vi "Begin.vi"(8 "error in":errorcluster) -> (0 "error out":errorcluster)   [LabVIEW 2018]
doc: "Called before other user functions, this VI is expected to open initial I/O refnums, load in file data, and do all program initialization. Notice that the <B>error out</B> terminal is simply used for data flow. Wiring it to other structures or subVIs ensures that this VI runs first."
uses:
  <vilib>/Rock Robotics/WPI/SafetyOutput/WPI_SafetyOutputConfigMenu.ctl
  <vilib>/Rock Robotics/WPI/DriverStation/WPI_DriverStationRobotMode2.ctl
  <vilib>/Rock Robotics/WPI/Joystick/WPI_JoystickDeviceEnum.ctl
  <vilib>/Rock Robotics/SystemInterfaces/DIO/FPGA_DIOChannel.ctl
  <vilib>/Rock Robotics/WPI/Solenoid/WPI_SolenoidChannel.ctl
  Robot Global Data.vi
  <vilib>/Rock Robotics/Network Tables/NT Write String Array.vi
  <vilib>/Rock Robotics/WPI/RobotDrive/WPI_RobotDriveOpen4MotorWithExistingMotors.vi
  <vilib>/Rock Robotics/WPI/Counter/WPI_CounterDigitalInputToDigitalSource.vi
  <vilib>/Rock Robotics/WPI/Counter/WPI_CounterOpen UpDown Mode.vi
  <vilib>/Rock Robotics/WPI/Solenoid/WPI_SolenoidOpenDouble.vi
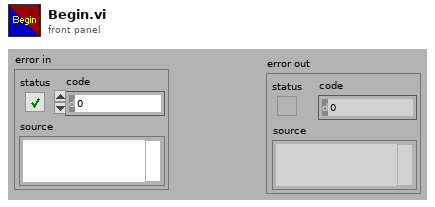
[diagram p1: front panel]
types:
  T1 = typedef "FPGA_DIOChannel.ctl" = enum8{"DIO 0", "DIO 1", "DIO 2", "DIO 3", "DIO 4", "DIO 5", "DIO 6", "DIO 7", "DIO 8", "DIO 9", "DIO MXP 0", "DIO MXP 1", "DIO MXP 2", "DIO MXP 3", "DIO MXP 4", "DIO MXP 5", "DIO MXP 6", "DIO MXP 7", "DIO MXP 8", "DIO MXP 9", "DIO MXP 10", "DIO MXP 11", "DIO MXP 12", "DIO MXP 13", "DIO MXP 14", "DIO MXP 15", "SPI Port CS1", "SPI Port CS2", "SPI Port CS3", "SPI Port MISO", "SPI Port MOSI", "Invalid"}
  T2 = typedef "WPI_SolenoidChannel.ctl" = enum8{"Solenoid 0", "Solenoid 1", "Solenoid 2", "Solenoid 3", "Solenoid 4", "Solenoid 5", "Solenoid 6", "Solenoid 7", "Invalid"}
  T3 = typedef "WPI_JoystickDeviceEnum.ctl" = enum16{"USB 0", "USB 1", "USB 2", "USB 3", "USB 4", "USB 5"}
  T4 = enum16{"Rising Edge", "Falling Edge", "Raising & Falling Edge", "Disabled"}
  T5 = typedef "WPI_DriverStationRobotMode2.ctl" = enum16{"Autonomous Disabled", "Autonomous Enabled", "Teleop Disabled", "Teleop Enabled", "Disconnected", "Finish", "Test Disabled", "Test Enabled", "Emergency Stopped"}
  T6 = typedef "WPI_SafetyOutputConfigMenu.ctl" = enum16{"Enable", "Disable"}
  T7 = typedef "WPI_MotorControlDeviceRef.ctl" = cluster{"DeviceStatus":errorcluster, "Type":T8, "PWM":cluster{"PWM Channel":T9, "DeadBand":T10}, "CAN":cluster{"Device Number":u8, "SetOutput VI Ref":variant, "GetOutput VI Ref":variant, "Enable VI Ref":variant, "Disable VI Ref":variant, "Data":variant}, "Invert":bool, "DIO PWM":cluster{"PWM \"Enable\" Channel":T9, "DIOChannel":T1, "PWM Rate":dbl}}
  T8 = typedef "WPI_MotorControlType.ctl" = enum16{"PWM", "CAN", "DIO PWM"}
  T9 = typedef "FPGA_DIOPWMChannel.ctl" = enum8{"PWM 0", "PWM 1", "PWM 2", "PWM 3", "PWM 4", "PWM 5", "PWM 6", "PWM 7", "PWM 8", "PWM 9", "PWM MXP 0", "PWM MXP 1", "PWM MXP 2", "PWM MXP 3", "PWM MXP 4", "PWM MXP 5", "PWM MXP 6", "PWM MXP 7", "PWM MXP 8", "PWM MXP 9", "Invalid"}
  T10 = typedef "WPI_PWMDeadband.ctl" = cluster{"Name":string, "maxPositivePwm":i32, "minPositivePwm":i32, "centerPwm":i32, "maxNegativePwm":i32, "minNegativePwm":i32, "angularRange":u16}
  T11 = typedef "WPI_DigitalInputDevRef.ctl" = cluster{"DevStatus":errorcluster, "DIO Channel":T1}
  T12 = typedef "WPI_DigitalOutputDevRef.ctl" = cluster{"DIO Channel":T1, "DevStatus":errorcluster}
  T13 = typedef "FPGA_CounterEncoderSourceConvertionLVSourceType.ctl" = cluster{"DevStatus":errorcluster, "AnalogTriggerMode?":bool, "DigitalMode":cluster{"DIO Channel":T14}, "AnalogTriggerMode":cluster{"AnalogTriggerIndex":T15, "OutputType":T16}}
  T14 = typedef "FPGA_DIODigitalSourceChannel.ctl" = enum8{"DIO 0", "DIO 1", "DIO 2", "DIO 3", "DIO 4", "DIO 5", "DIO 6", "DIO 7", "DIO 8", "DIO 9", "DIO MXP 0", "DIO MXP 1", "DIO MXP 2", "DIO MXP 3", "DIO MXP 4", "DIO MXP 5", "DIO MXP 6", "DIO MXP 7", "DIO MXP 8", "DIO MXP 9", "DIO MXP 10", "DIO MXP 11", "DIO MXP 12", "DIO MXP 13", "DIO MXP 14", "DIO MXP 15", "SPI Port CS1", "SPI Port CS2", "SPI Port CS3", "SPI Port MISO", "SPI Port MOSI", "Disabled"}
  T15 = typedef "FPGA_AnalogTriggerIndex.ctl" = enum8{"Trig 0", "Trig 1", "Trig 2", "Trig 3", "Trig 4", "Trig 5", "Trig 6", "Trig 7", "Invalid"}
  T16 = typedef "FPGA_AnalogTriggerOutType.ctl" = enum16{"InWindow", "TriggerState", "Rising", "Falling"}
  T17 = typedef "WPI_EncoderDevRef.ctl" = cluster{"DevStatus":errorcluster, "EncoderIndex":T18, "CounterIndex":T19, "DistancePerCount":dbl, "Decoding Type":T20}
  T18 = typedef "FPGA_EncoderIdx.ctl" = enum8{"Enc 0", "Enc 1", "Enc 2", "Enc 3", "Enc 4", "Enc 5", "Enc 6", "Enc 7", "Invalid"}
  T19 = typedef "FPGA_CounterCtrSystemIndex.ctl" = enum8{"Ctr 0", "Ctr 1", "Ctr 2", "Ctr 3", "Ctr 4", "Ctr 5", "Ctr 6", "Ctr 7", "Invalid"}
  T20 = typedef "WPI_EncoderType.ctl" = enum16{"1x", "2x", "4x"}
  T21 = typedef "WPI_RobotDriveDevRef.ctl" = cluster{"DevStatus":errorcluster, "Motors[]":T7[], "Square Inputs":bool, "Max Output":dbl}
  T22 = typedef "WPI_JoystickDevRef.ctl" = cluster{"Device":T3}
  T23 = typedef "WPI_SolenoidDevRef.ctl" = cluster{"DevStatus":errorcluster, "Pneumatics Control Module":u8, "Forward Solenoid Channel":T2, "Reverse Solenoid Channel":T2}
  T24 = typedef "WPI_CounterDevRef.ctl" = cluster{"DevStatus":errorcluster, "CntIndex":T19}
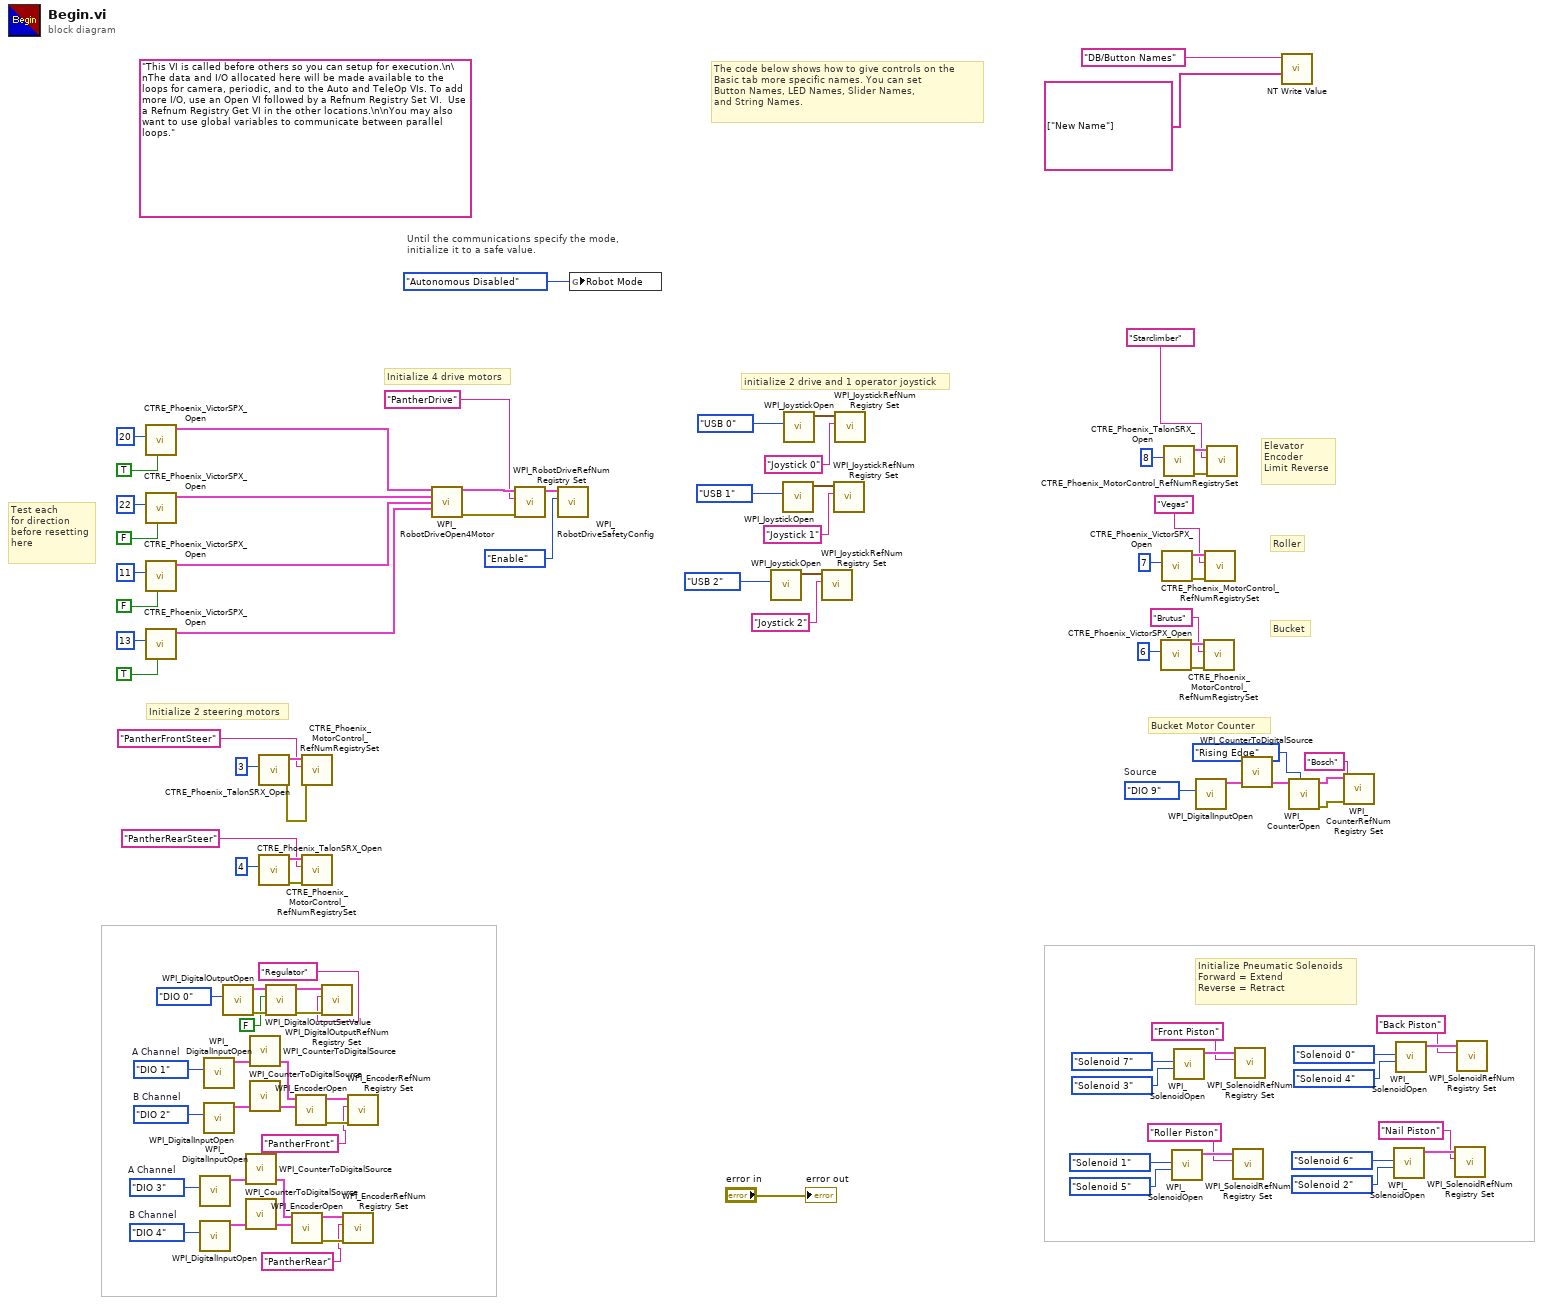
[diagram p0: block diagram]
diagram:
  w32 = FPGA_DIOChannel."DIO 9"  # Source
  w57 = FPGA_DIOChannel."DIO 4"  # B Channel
  w56 = FPGA_DIOChannel."DIO 3"  # A Channel
  w63 = FPGA_DIOChannel."DIO 2"  # B Channel
  w62 = FPGA_DIOChannel."DIO 1"  # A Channel
  (unwired) "This VI is called before others so you can setup for execution.\n\nThe data and I/O allocated here will be made available to the loops for camera, periodic, and to the Auto and TeleOp VIs. To add more I/O, use an Open VI followed by a Refnum Registry Set VI.  Use a Refnum Registry Get VI in the other locations.\n\nYou may also want to use global variables to communicate between parallel loops."
  # "Test each\nfor direction\nbefore resetting\nhere"
  # "Initialize Pneumatic Solenoids\nForward = Extend\nReverse = Retract"
  # "Initialize 2 steering motors"
  # "Bucket Motor Counter"
  # "Bucket"
  # "Roller"
  # "Elevator\nEncoder\nLimit Reverse"
  # "The code below shows how to give controls on the\nBasic tab more specific names. You can set\nButton Names, LED Names, Slider Names,\nand String Names."
  # "initialize 2 drive and 1 operator joystick"
  # "Until the communications specify the mode,\ninitialize it to a safe value."
  # "Initialize 4 drive motors"
  n1 = call <vilib>:"CTRE_Phoenix_VictorSPX_Open.vi"("Invert"=TRUE, "Device Number"=u8 20) -> ("CAN Talon SRX Ref"=w81:T7)  [unwired: 8 in, 1 out]
  n2 = call <vilib>:"CTRE_Phoenix_VictorSPX_Open.vi"("Invert"=FALSE, "Device Number"=u8 22) -> ("CAN Talon SRX Ref"=w78:T7)  [unwired: 8 in, 1 out]
  n3 = call <vilib>:"CTRE_Phoenix_VictorSPX_Open.vi"("Invert"=FALSE, "Device Number"=u8 11) -> ("CAN Talon SRX Ref"=w75:T7)  [unwired: 8 in, 1 out]
  n4 = call <vilib>:"CTRE_Phoenix_VictorSPX_Open.vi"("Invert"=TRUE, "Device Number"=u8 13) -> ("CAN Talon SRX Ref"=w72:T7)  [unwired: 8 in, 1 out]
  n5 = call <vilib>:"WPI_DigitalInputOpen.vi"("DIO Channel"=w56) -> ("DigitalInputDevRef"=w53:T11)  [unwired: 1 in, 9 out]
  n6 = call <vilib>:"WPI_DigitalInputOpen.vi"("DIO Channel"=w57) -> ("DigitalInputDevRef"=w54:T11)  [unwired: 1 in, 9 out]
  n7 = call <vilib>:"WPI_DigitalInputOpen.vi"("DIO Channel"=w62) -> ("DigitalInputDevRef"=w59:T11)  [unwired: 1 in, 9 out]
  n8 = call <vilib>:"WPI_DigitalInputOpen.vi"("DIO Channel"=w63) -> ("DigitalInputDevRef"=w60:T11)  [unwired: 1 in, 9 out]
  n9 = call <vilib>:"WPI_DigitalOutputOpen.vi"("DIO Channel"=FPGA_DIOChannel."DIO 0") -> ("error out"=w3:errorcluster, "DigitalOutputDevRef"=w6:T12)  [unwired: 9 in]
  n10 = call-poly <vilib>:"WPI_CounterToDigitalSource.vi"("DigitalInputDevRef"=w53) -> ("Digital Source"=w52:T13)  [unwired: 6 out]
  n11 = call-poly <vilib>:"WPI_CounterToDigitalSource.vi"("DigitalInputDevRef"=w54) -> ("Digital Source"=w55:T13)  [unwired: 6 out]
  n12 = call-poly <vilib>:"WPI_CounterToDigitalSource.vi"("DigitalInputDevRef"=w59) -> ("Digital Source"=w58:T13)  [unwired: 6 out]
  n13 = call-poly <vilib>:"WPI_CounterToDigitalSource.vi"("DigitalInputDevRef"=w60) -> ("Digital Source"=w61:T13)  [unwired: 6 out]
  n14 = call <vilib>:"CTRE_Phoenix_TalonSRX_Open.vi"("Device Number"=u8 3) -> ("error out"=w70:errorcluster, "CAN Talon SRX Ref"=w71:T7)  [unwired: 9 in]
  n15 = call <vilib>:"CTRE_Phoenix_TalonSRX_Open.vi"("Device Number"=u8 4) -> ("error out"=w65:errorcluster, "CAN Talon SRX Ref"=w66:T7)  [unwired: 9 in]
  n16 = call <vilib>:"WPI_DigitalOutputSetValue.vi"("error in (no error)"=w3, "Value"=FALSE, "DigitalOutputDevRef"=w6) -> ("error out"=w4:errorcluster, "DigitalOutputDevRef"=w5:T12)  [unwired: 7 in]
  n17 = call <vilib>:"WPI_EncoderOpen.vi"("BSource"=w55, "ASource"=w52) -> ("error out"=w49:errorcluster, "EncoderDevRef"=w48:T17)  [unwired: 6 in, 2 out]
  n18 = call <vilib>:"WPI_EncoderOpen.vi"("BSource"=w61, "ASource"=w58) -> ("error out"=w51:errorcluster, "EncoderDevRef"=w50:T17)  [unwired: 6 in, 2 out]
  n19 = call <vilib>:"CTRE_Phoenix_MotorControl_RefNumRegistrySet.vi"("error in (no error)"=w70, "refnum name"="PantherFrontSteer", "PhoenixMotorControlDevRef"=w71) -> ()  [unwired: 7 in, 2 out]
  n20 = call <vilib>:"CTRE_Phoenix_MotorControl_RefNumRegistrySet.vi"("error in (no error)"=w65, "refnum name"="PantherRearSteer", "PhoenixMotorControlDevRef"=w66) -> ()  [unwired: 7 in, 2 out]
  n21 = call <vilib>:"WPI_DigitalOutputRefNum Registry Set.vi"("error in (no error)"=w4, "refnum name"="Regulator", "DigitalOutputDevRef"=w5) -> ()  [unwired: 7 in, 2 out]
  n22 = call <vilib>:"WPI_EncoderRefNum Registry Set.vi"("error in (no error)"=w49, "refnum name"="PantherRear", "EncoderDevRef"=w48) -> ()  [unwired: 7 in, 2 out]
  n23 = call <vilib>:"WPI_EncoderRefNum Registry Set.vi"("error in (no error)"=w51, "refnum name"="PantherFront", "EncoderDevRef"=w50) -> ()  [unwired: 7 in, 2 out]
  n24 = call-poly <vilib>:"WPI_RobotDriveOpen4Motor.vi"("Rear Left Motor Dev Ref"=w81, "Rear Right Motor Dev Ref"=w78, "Front Left Motor Dev Ref"=w75, "Front Right Motor Dev Ref"=w72) -> ("RobotDriveDevRef"=w84:T21, "error out"=w85:errorcluster)  [unwired: 10 in]
  n25 = call <vilib>:"WPI_RobotDriveRefNum Registry Set.vi"("error in (no error)"=w85, "refnum name"="PantherDrive", "RobotDriveDevRef"=w84) -> ("RobotDriveDevRef"=w82:T21)  [unwired: 7 in, 1 out]
  n26 = call <vilib>:"WPI_RobotDriveSafetyConfig.vi"("mode"=WPI_SafetyOutputConfigMenu."Enable", "RobotDriveDevRef"=w82) -> ()  [unwired: 8 in, 2 out]
  n27 = global write "Robot Global Data.vi" "Robot Mode"(WPI_DriverStationRobotMode2."Autonomous Disabled" ("Robot Mode")) -> ()
  n28 = call <vilib>:"WPI_JoystickOpen.vi"("JoystickDevice"=WPI_JoystickDeviceEnum."USB 2") -> ("JoystickDevRef"=w25:T22)  [unwired: 10 in]
  n29 = call <vilib>:"WPI_JoystickOpen.vi"("JoystickDevice"=WPI_JoystickDeviceEnum."USB 1") -> ("JoystickDevRef"=w89:T22)  [unwired: 10 in]
  n30 = call <vilib>:"WPI_JoystickOpen.vi"("JoystickDevice"=WPI_JoystickDeviceEnum."USB 0") -> ("JoystickDevRef"=w95:T22)  [unwired: 10 in]
  n31 = call <vilib>:"WPI_JoystickRefNum Registry Set.vi"("refnum name"="Joystick 2", "JoystickDevRef"=w25) -> ()  [unwired: 8 in, 2 out]
  n32 = call <vilib>:"WPI_JoystickRefNum Registry Set.vi"("refnum name"="Joystick 1", "JoystickDevRef"=w89) -> ()  [unwired: 8 in, 2 out]
  n33 = call <vilib>:"WPI_JoystickRefNum Registry Set.vi"("refnum name"="Joystick 0", "JoystickDevRef"=w95) -> ()  [unwired: 8 in, 2 out]
  n34 = call <vilib>:"CTRE_Phoenix_VictorSPX_Open.vi"("Device Number"=u8 6) -> ("error out"=w43:errorcluster, "CAN Talon SRX Ref"=w44:T7)  [unwired: 9 in]
  n35 = call <vilib>:"CTRE_Phoenix_VictorSPX_Open.vi"("Device Number"=u8 7) -> ("error out"=w35:errorcluster, "CAN Talon SRX Ref"=w36:T7)  [unwired: 9 in]
  n36 = call <vilib>:"CTRE_Phoenix_TalonSRX_Open.vi"("Device Number"=u8 8) -> ("error out"=w39:errorcluster, "CAN Talon SRX Ref"=w40:T7)  [unwired: 9 in]
  n37 = call-poly <vilib>:"WPI_SolenoidOpen.vi"("Reverse Solenoid Channel"=WPI_SolenoidChannel."Solenoid 5", "Forward Solenoid Channel"=WPI_SolenoidChannel."Solenoid 1") -> ("SolenoidDevRef"=w19:T23)  [unwired: 8 in, 1 out]
  n38 = call-poly <vilib>:"WPI_SolenoidOpen.vi"("Reverse Solenoid Channel"=WPI_SolenoidChannel."Solenoid 3", "Forward Solenoid Channel"=WPI_SolenoidChannel."Solenoid 7") -> ("SolenoidDevRef"=w15:T23)  [unwired: 8 in, 1 out]
  n39 = call <vilib>:"WPI_DigitalInputOpen.vi"("DIO Channel"=w32) -> ("DigitalInputDevRef"=w31:T11)  [unwired: 1 in, 9 out]
  n40 = call <vilib>:"CTRE_Phoenix_MotorControl_RefNumRegistrySet.vi"("error in (no error)"=w43, "refnum name"="Brutus", "PhoenixMotorControlDevRef"=w44) -> ()  [unwired: 7 in, 2 out]
  n41 = call <vilib>:"CTRE_Phoenix_MotorControl_RefNumRegistrySet.vi"("error in (no error)"=w35, "refnum name"="Vegas", "PhoenixMotorControlDevRef"=w36) -> ()  [unwired: 7 in, 2 out]
  n42 = call <vilib>:"CTRE_Phoenix_MotorControl_RefNumRegistrySet.vi"("error in (no error)"=w39, "refnum name"="Starclimber", "PhoenixMotorControlDevRef"=w40) -> ()  [unwired: 7 in, 2 out]
  n43 = call <vilib>:"WPI_SolenoidRefNum Registry Set.vi"("refnum name"="Roller Piston", "SolenoidDevRef"=w19) -> ()  [unwired: 8 in, 2 out]
  n44 = call <vilib>:"WPI_SolenoidRefNum Registry Set.vi"("refnum name"="Front Piston", "SolenoidDevRef"=w15) -> ()  [unwired: 8 in, 2 out]
  n45 = call-poly <vilib>:"WPI_CounterToDigitalSource.vi"("DigitalInputDevRef"=w31) -> ("Digital Source"=w33:T13)  [unwired: 6 out]
  n46 = call-poly <vilib>:"NT Write Value.vi"("String Array"=string[] ["New Name"], "Name"="DB/Button Names") -> ()  [unwired: 9 in, 1 out]
  n47 = call-poly <vilib>:"WPI_CounterOpen.vi"("UpEdge"=T4."Rising Edge", "Up Source"=w33) -> ("error out"=w30:errorcluster, "CounterDevRef"=w29:T24)  [unwired: 5 in, 3 out]
  n48 = call <vilib>:"WPI_CounterRefNum Registry Set.vi"("error in (no error)"=w30, "refnum name"="Bosch", "CounterDevRef"=w29) -> ()  [unwired: 7 in, 2 out]
  n49 = call-poly <vilib>:"WPI_SolenoidOpen.vi"("Reverse Solenoid Channel"=WPI_SolenoidChannel."Solenoid 2", "Forward Solenoid Channel"=WPI_SolenoidChannel."Solenoid 6") -> ("SolenoidDevRef"=w11:T23)  [unwired: 8 in, 1 out]
  n50 = call-poly <vilib>:"WPI_SolenoidOpen.vi"("Reverse Solenoid Channel"=WPI_SolenoidChannel."Solenoid 4", "Forward Solenoid Channel"=WPI_SolenoidChannel."Solenoid 0") -> ("SolenoidDevRef"=w23:T23)  [unwired: 8 in, 1 out]
  n51 = call <vilib>:"WPI_SolenoidRefNum Registry Set.vi"("refnum name"="Nail Piston", "SolenoidDevRef"=w11) -> ()  [unwired: 8 in, 2 out]
  n52 = call <vilib>:"WPI_SolenoidRefNum Registry Set.vi"("refnum name"="Back Piston", "SolenoidDevRef"=w23) -> ()  [unwired: 8 in, 2 out]
  "error out" <- "error in"
